vi "Two Sessions Two Pins Two Instruments One Site.vi"(8 "error in":errorcluster) -> (0 "error out":errorcluster, 3 "data out":T1)   [LabVIEW 2020, in "MeasurementServerTests.lvlib"]
uses:
  MeasurementServerTests.lvlib
  Runtime/MeasurementLink Session Management/Session Reservation/Data.ctl
  Runtime/MeasurementLink Session Management/Session Reservation/Session and Driver Info.ctl
  Runtime/MeasurementLink Session Management Client/RPC Messages/ni_measurementlink_sessionmanagement_v1_SessionInformation.ctl
  Runtime/MeasurementLink Session Management Client/RPC Messages/nidevice_grpc_Session.ctl
  Runtime/MeasurementLink Session Management Client/RPC Messages/ni_measurementlink_sessionmanagement_v1_ChannelMapping.ctl
  Runtime/MeasurementLink Session Management Client/MeasurementLink Session Management Client.lvlib
  Runtime/MeasurementLink Session Management/Session Reservation/Session Reservation.lvclass
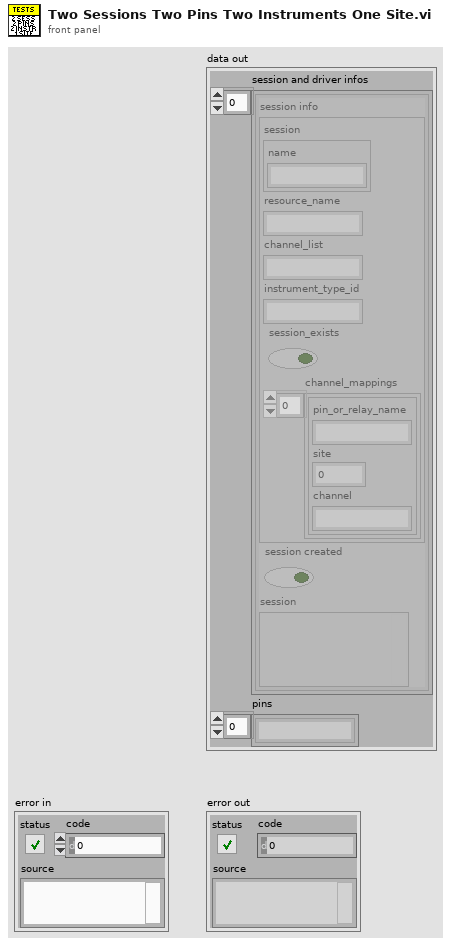
[diagram p1: front panel]
types:
  T1 = typedef "MeasurementLink Session Management.lvlib/Session Reservation.lvclass/Data.ctl" = cluster{"session and driver infos":T2[], "pins":string[]}
  T2 = typedef "MeasurementLink Session Management.lvlib/Session Reservation.lvclass/Session and Driver Info.ctl" = cluster{"session info":T3, "session created":bool, "session":variant}
  T3 = typedef "MeasurementLink Session Management Client.lvlib/ni_measurementlink_sessionmanagement_v1_SessionInformation.ctl" = cluster{"session":T4, "resource_name":string, "channel_list":string, "instrument_type_id":string, "session_exists":bool, "channel_mappings":T5[]}
  T4 = typedef "MeasurementLink Session Management Client.lvlib/nidevice_grpc_Session.ctl" = cluster{"name":string}
  T5 = typedef "MeasurementLink Session Management Client.lvlib/ni_measurementlink_sessionmanagement_v1_ChannelMapping.ctl" = cluster{"pin_or_relay_name":string, "site":i32, "channel":string}
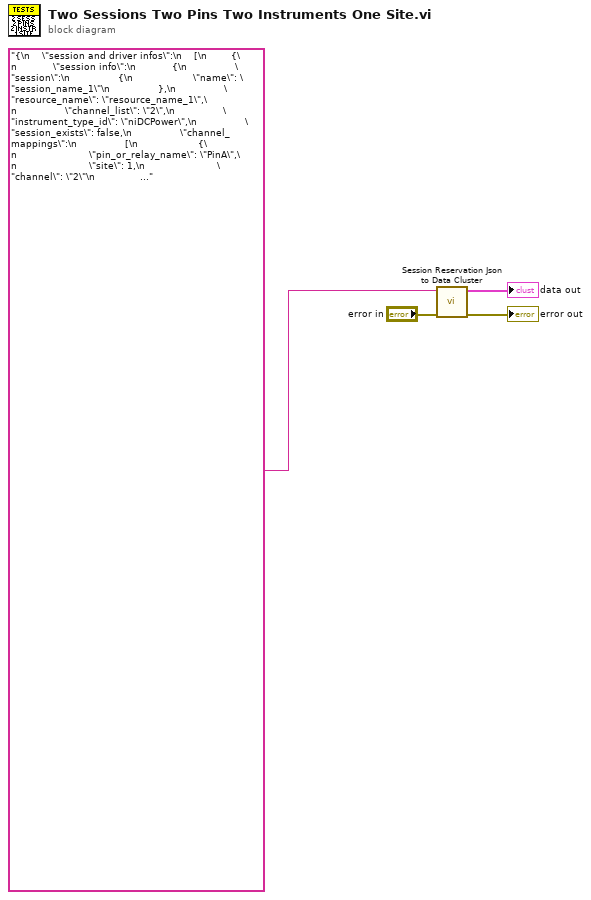
[diagram p0: block diagram]
diagram:
  n1 = call "Session Reservation Json to Data Cluster.vi"("error in"="error in", "json in"="{\n    \"session and driver infos\":\n    [\n        {\n            \"session info\":\n            {\n                \"session\":\n                {\n                    \"name\": \"session_name_1\"\n                },\n                \"resource_name\": \"resource_name_1\",\n                \"channel_list\": \"2\",\n                \"instrument_type_id\": \"niDCPower\",\n                \"session_exists\": false,\n                \"channel_mappings\":\n                [\n                    {\n                        \"pin_or_relay_name\": \"PinA\",\n                        \"site\": 1,\n                        \"channel\": \"2\"\n                    }\n                ]\n            },\n            \"session created\": false,\n            \"session\": \"\"\n        },\n        {\n            \"session info\":\n            {\n                \"session\":\n                {\n                    \"name\": \"session_name_2\"\n                },\n                \"resource_name\": \"resource_name_2\",\n                \"channel_list\": \"4\",\n                \"instrument_type_id\": \"niFgen\",\n                \"session_exists\": false,\n                \"channel_mappings\":\n                [\n                    {\n                        \"pin_or_relay_name\": \"PinB\",\n                        \"site\": 1,\n                        \"channel\": \"4\"\n                    }\n                ]\n            },\n            \"session created\": false,\n            \"session\": \"\"\n        }\n    ],\n    \"pins\":\n    [\n        \"PinA\",\n        \"PinB\"\n    ]\n}") -> ("error out"=→"error out":errorcluster, "data out"=→"data out":T1)  [unwired: 8 in]
